vi "Camera module.vi"(8 "error in (no error)":errorcluster) -> (0 "error out":errorcluster)   [LabVIEW 2016]
uses:
  <vilib>/vision/Image Controls.llb/IMAQ Image.ctl
  <vilib>/userdefined/High Color/IMAQdx.ctl
  General/Controls/Queue modes.ctl
  General/Controls/staus modes.ctl
  Controls/Camera queue.ctl
  Controls/Camera states.ctl
  <vilib>/vision/driver/NI_Vision_Acquisition_Software.lvlib
panel:
  out "error out 2":errorcluster
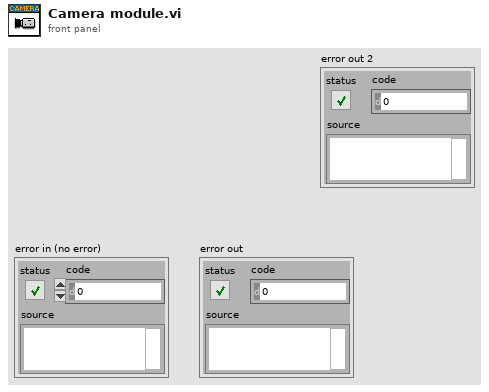
[diagram p1: front panel]
types:
  T1 = typedef "Queue modes.ctl" = enum16{"Initialise", "Destroy", "Get"}
  T2 = typedef "IMAQdx.ctl" = refnum<k21>
  T3 = typedef "IMAQ Image.ctl" = refnum<image>
  T4 = typedef "References.ctl" = cluster{"Tab Control":refnum<vi>, "Logo 1":refnum<vi>, "Logo 2":refnum<vi>, "Connect Actuator":refnum<vi>, "LIVE DATA":refnum<vi>, "Speed":refnum<vi>, "Home position":refnum<vi>, "Limit position":refnum<vi>, "Trigger":refnum<vi>, "Current position":refnum<vi>, "Connect Camera":refnum<vi>, "TEST DATA":refnum<vi>, "LIVE DATA Force":refnum<vi>, "Connect DAQ":refnum<vi>, "Initialised":refnum<vi>, "Test":refnum<vi>}
  T5 = typedef "Camera queue.ctl" = cluster{"State":T6, "Data":variant}
  T6 = typedef "Camera states.ctl" = enum16{"Initialise", "Setup", "Connect", "Snap", "Close", "Shutdown"}
  T7 = enum32{"Invalid", "Standard", "Closed", "Hidden", "Minimized", "Maximized"}
  T8 = enum8{"Enabled", "Disabled", "Disabled and Grayed Out"}
  T9 = typedef "staus modes.ctl" = enum16{"Status", "Testing", "Webcam", "DAQ", "Actuator", "Initialise"}
  T10 = cluster{"Type":u32, "Version":u32, "Flags":u32, "SerialNumberHigh":u32, "SerialNumberLow":u32, "BusType":u32, "InterfaceName":string, "VendorName":string, "ModelName":string, "CameraFileName":string, "CameraAttributeURL":string}[]
  T11 = typedef "Test settings.ctl" = cluster{"Speed (mm/s)":dbl, "Position limit":bool, "Position limit (mm)":dbl, "Load limit":bool, "Load limit (N)":dbl, "No. of repeats":u16, "Test identifier":string, "Time wait":bool, "Wait time (s)":dbl, "Trigger wait":bool, "Send trigger":bool, "Test notes":string, "Snap intervals":bool, "Time interval (s)":dbl}
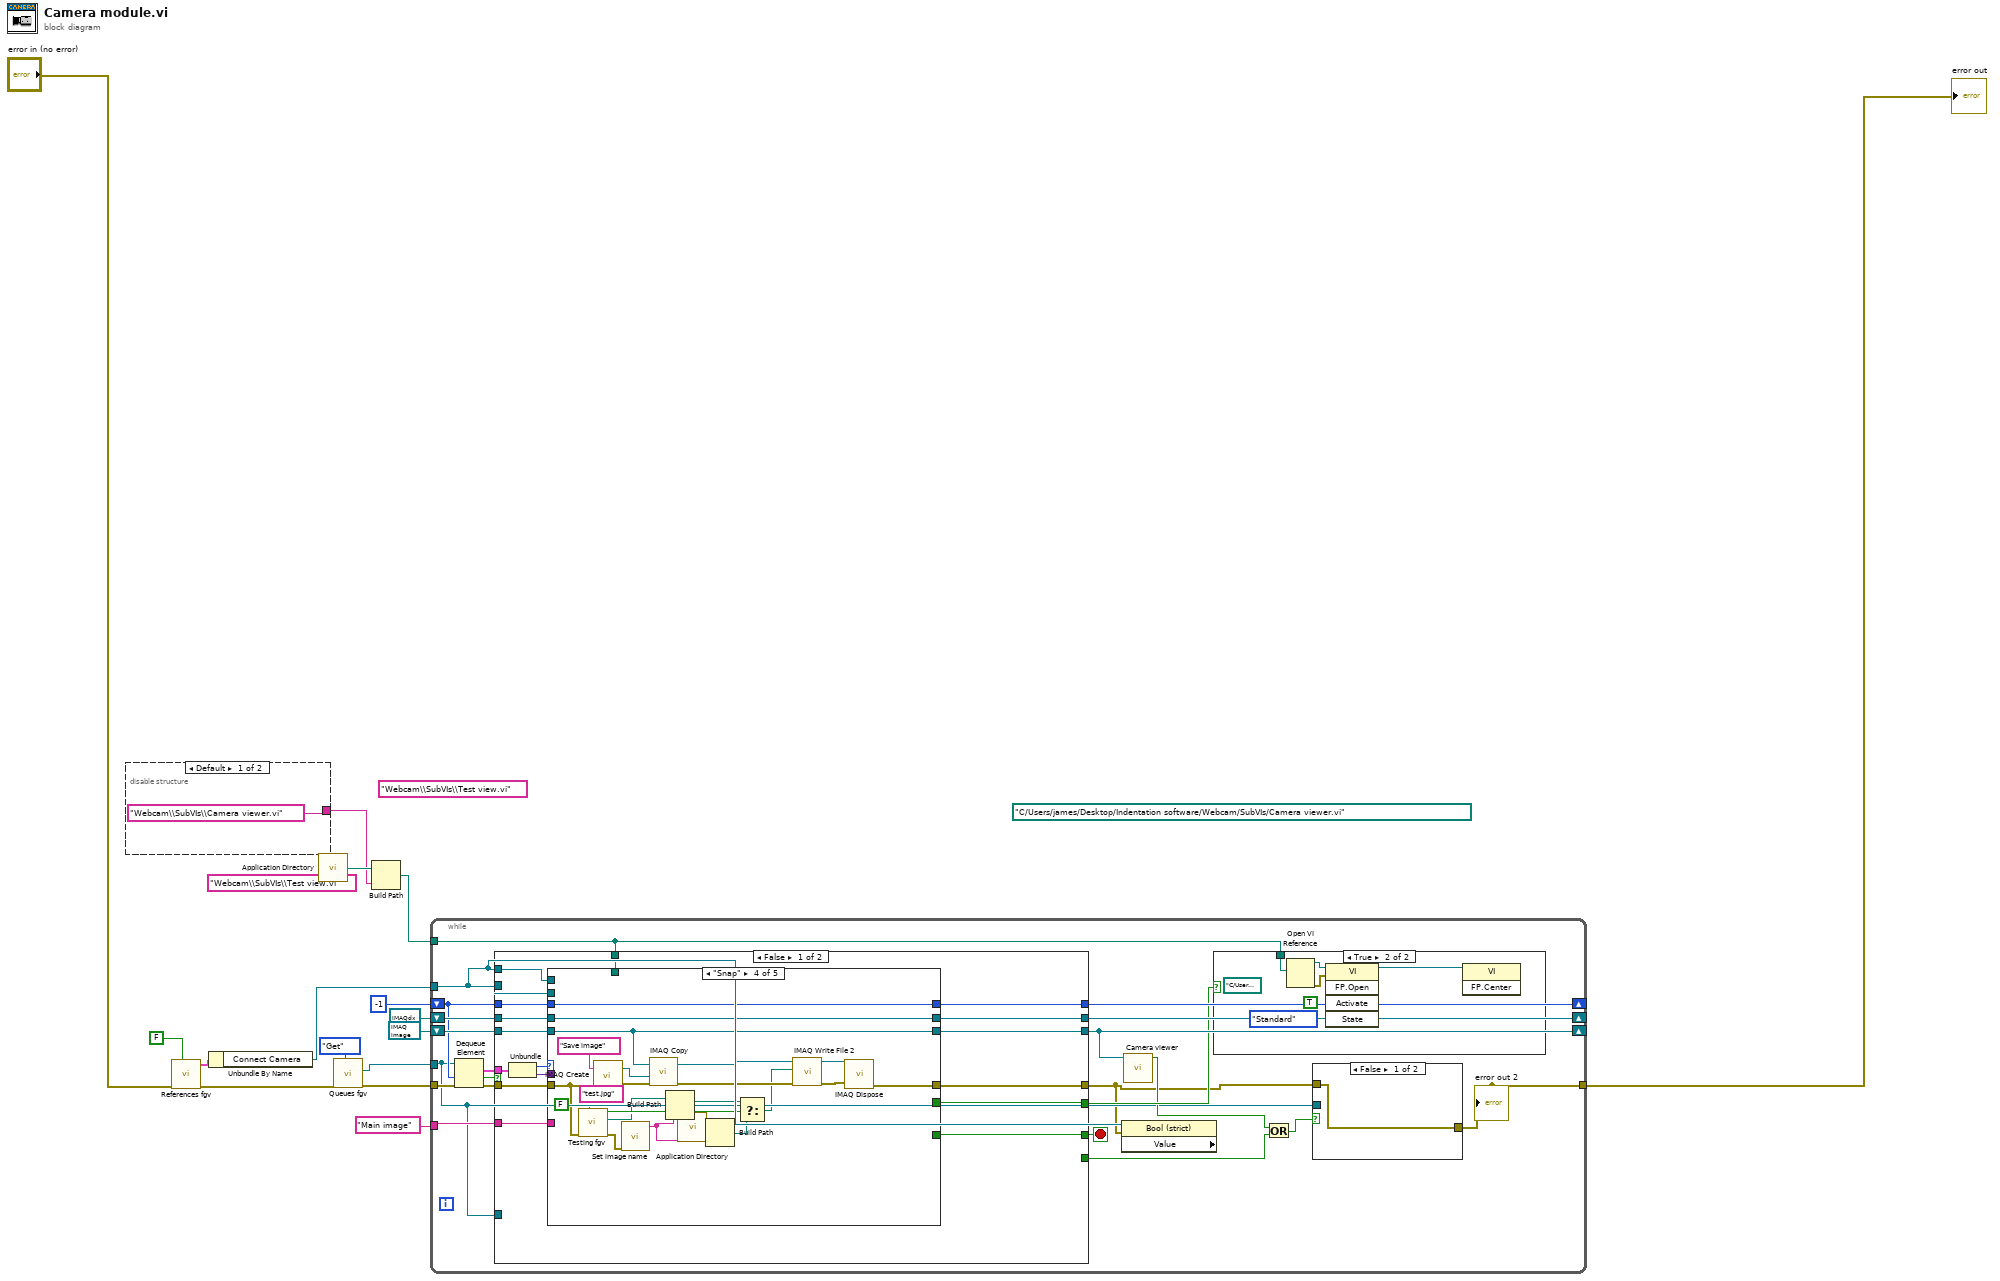
[diagram p0: block diagram]
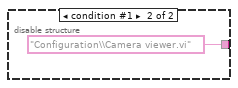
[diagram p2: hidden frame]
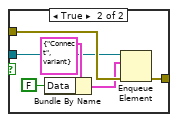
[diagram p3: hidden frame]
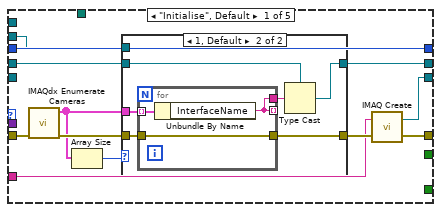
[diagram p5: hidden frame]
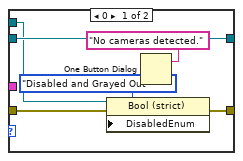
[diagram p6: hidden frame]
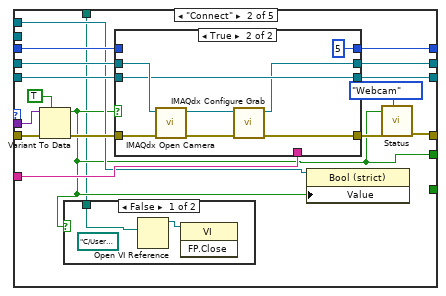
[diagram p7: hidden frame]
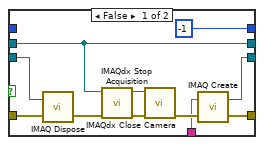
[diagram p9: hidden frame]
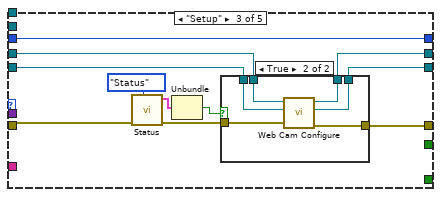
[diagram p10: hidden frame]
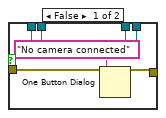
[diagram p11: hidden frame]
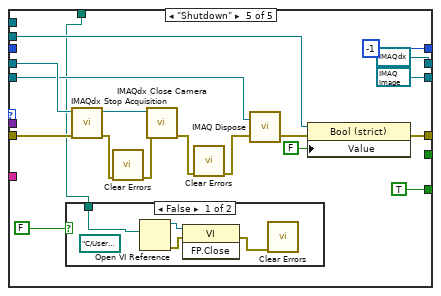
[diagram p12: hidden frame]
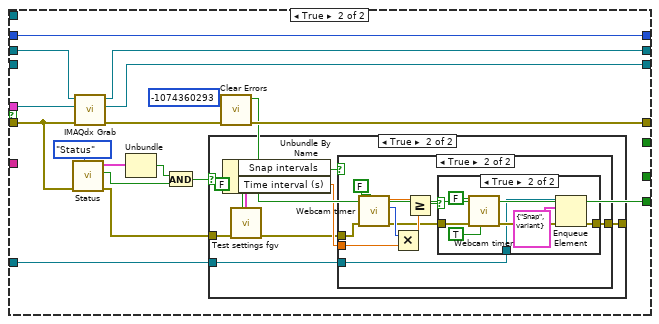
[diagram p14: hidden frame]
diagram:
  (unwired) "Webcam\\SubVIs\\Test view.vi" ("name or relative path")
  (unwired) "Webcam\\SubVIs\\Test view.vi" ("name or relative path")
  (unwired) path "C:/Users/james/Desktop/Indentation software/Webcam/SubVIs/Camera viewer.vi" ("vi path")
  n1 = disable-structure shown="Default" {
    disable-tunnel: ["Webcam\\SubVIs\\Camera viewer.vi" ("name or relative path") "Configuration\\Camera viewer.vi" ("name or relative path")] -> w1
    frame condition #0 (active) {
    }
    frame condition #1 {
    }
  }
  n2 = call "References fgv.vi"("Set?"=FALSE, "error in (no error)"="error in (no error)") -> ("error out"=w8:errorcluster, "Cluster"=w5:T4)  [unwired: 8 in]
  n3 = Unbundle By Name(w5) -> ("Connect Camera"=w4:refnum<vi>)
  n4 = call <vilib>:"Application Directory.vi"() -> ("Application Directory"=w3:path)
  n5 = call "Queues fgv.vi"("Modes"=Queue_modes."Get", "error in (no error)"=w8) -> ("error in (no error) 2"=w15:errorcluster, "Camera"=w14:refnum<queue>)  [unwired: 6 in, 2 out]
  n6 = Build Path(base path=w3, name or relative path=w1) -> (appended path=w2:path)
  n7 = while {
    tunnel: w14 -> [w21]
    tunnel: w15 -> [w39]
    tunnel: [w26] -> w13
    shift-right: [w33] -> _
    shift-left: T2 refnum ("Session Out") -> [w34]
    shift-right: [w28] -> _
    shift-left: T3 refnum ("New Image") -> [w35]
    tunnel: w4 -> [w22]
    shift-right: [w30] -> _
    shift-left: -1 ("timeout in ms (-1)") -> [w31]
    tunnel: "Main image" ("Image Name") -> [w29]
    tunnel: w2 -> [w20]
    stop <- w36 stop-if-true
    n8 = Dequeue Element(queue=w21, timeout in ms (-1)=w31, error in (no error)=w39) -> (element=w38:T5, timed out?=w32:bool, error out=w37:errorcluster)  [unwired: 1 out]
    n9 = case shown="False" w32 {
      tunnel: w38 -> [w69 _]
      tunnel: w37 -> [w68 w206]
      tunnel: [w65 _] -> w36
      tunnel: [w64 w209] -> w19
      tunnel: [w63 w212] -> w28
      tunnel: w35 -> [w62 w214]
      tunnel: w22 -> [w61 _]
      tunnel: w34 -> [w60 w215]
      tunnel: [w59 w213] -> w33
      tunnel: w31 -> [w58 w211]
      tunnel: [w57 w211] -> w30
      tunnel: w29 -> [w56 _]
      tunnel: [w55 _] -> w27
      tunnel: w22 -> [w54 _]
      tunnel: [_ w207] -> w24
      tunnel: w20 -> [w53 _]
      tunnel: w21 -> [_ w199]
      frame False {
        n10 = Unbundle(w69) -> ("State"=w67:T6, "Data"=w66:variant)
        n11 = case shown="\"Snap\"" w67 {
          tunnel: w68 -> [w76 w113 w139 w157 w189]
          tunnel: w66 -> [_ w112 _ _ _]
          tunnel: [_ _ _ _ TRUE] -> w65
          tunnel: [w81 w100 w145 w168 w193] -> w64
          tunnel: [w80 w107 w141 w171 T3 refnum ("New Image out")] -> w63
          tunnel: w62 -> [_ w108 w143 w171 w187]
          tunnel: w61 -> [w71 _ _ _ w191]
          tunnel: w60 -> [w78 w109 w144 w176 w188]
          tunnel: [w77 w106 w142 w176 T2 refnum ("Session Out out")] -> w59
          tunnel: w58 -> [w79 w105 w140 w175 _]
          tunnel: [w79 w104 w140 w175 -1 ("timeout in ms (-1)")] -> w57
          tunnel: w56 -> [w73 w103 _ _ _]
          tunnel: [_ w98 _ _ _] -> w55
          tunnel: w54 -> [_ w99 _ _ _]
          tunnel: w53 -> [_ w97 _ _ w178]
          frame "Initialise", Default {
            n12 = call <vilib>:"IMAQdx Enumerate Cameras.vi"("error in"=w76) -> ("error out"=w75:errorcluster, "Camera Information Array"=w72:T10)  [unwired: 9 in]
            n13 = Array Size(array=w72) -> (size(s)=w70:i32)
            n14 = case shown="1, Default" w70 {
              tunnel: w78 -> [w87 w93]
              tunnel: [w87 w92] -> w77
              tunnel: w75 -> [w85 w91]
              tunnel: [w83 w89] -> w74
              tunnel: w72 -> [_ w88]
              tunnel: w71 -> [w84 _]
              frame 0 {
                n15 = property class="Bool (strict)"(reference=w84, error in=w85, "DisabledEnum"=T8."Disabled and Grayed Out" ("Disabled")) -> (error out=w83:errorcluster)  [unwired: 1 out]
                n16 = One Button Dialog(message="No cameras detected.") -> ()  [unwired: 1 in, 1 out]
              }
              frame 1, Default {
                n17 = for {
                  tunnel: w88 -> [w96] mode=indexing
                  tunnel: [w95] -> _ mode=indexing
                  tunnel: [w95] -> w90
                  tunnel: w91 -> [w94]
                  tunnel: [w94] -> w89
                  n18 = Unbundle By Name(w96) -> ("InterfaceName"=w95:string)
                }
                n19 = Type Cast(type=w93, x=w90) -> (*(type *) &x=w92:T2)
              }
            }
            n20 = call "IMAQ Create"("Image Name"=w73, "error in (no error)"=w74) -> ("New Image"=w80:T3, "error out"=w81:errorcluster)  [unwired: 3 in]
          }
          frame "Connect" {
            n21 = Variant To Data(error in=w113, type=TRUE, Variant=w112) -> (data=w98:bool, error out=w110:errorcluster)
            n22 = case shown="False" w98 {
              tunnel: w97 -> [w114 _]
              frame False {
                (unwired) path "C:/Users/james/Desktop/Indentation software/Webcam/SubVIs/Camera viewer.vi" ("vi path")
                n23 = Open VI Reference(vi path=w114) -> (vi reference=w115:refnum<vi>)  [unwired: 5 in, 1 out]
                n24 = invoke class="VI" method="FP.Close"(reference=w115) -> ()  [unwired: 2 in, 3 out]
              }
              frame True {
              }
            }
            n25 = case shown="True" w98 {
              tunnel: w110 -> [w122 w134]
              tunnel: w109 -> [w123 w133]
              tunnel: w108 -> [w120 w132]
              tunnel: [w118 w128] -> w102
              tunnel: [w117 w132] -> w107
              tunnel: [w123 w127] -> w106
              tunnel: w105 -> [_ _]
              tunnel: [-1 ("timeout in ms (-1)") 5 ("timeout in ms (-1)")] -> w104
              tunnel: w103 -> [w116 _]
              frame False {
                n26 = call "IMAQ Dispose"("Image"=w120, "error in (no error)"=w122) -> ("error out"=w121:errorcluster)  [unwired: 4 in]
                n27 = call <vilib>:"IMAQdx Stop Acquisition.vi"("error in"=w121, "Session In"=w123) -> ("error out"=w125:errorcluster, "Session Out"=w126:T2)  [unwired: 8 in]
                n28 = call <vilib>:"IMAQdx Close Camera.vi"("error in"=w125, "Session In"=w126) -> ("error out"=w119:errorcluster)  [unwired: 9 in]
                n29 = call "IMAQ Create"("Image Name"=w116, "error in (no error)"=w119) -> ("New Image"=w117:T3, "error out"=w118:errorcluster)  [unwired: 3 in]
              }
              frame True {
                n30 = call <vilib>:"IMAQdx Open Camera.vi"("error in"=w134, "Session In"=w133) -> ("error out"=w129:errorcluster, "Session Out"=w130:T2)  [unwired: 1 in, 7 out]
                n31 = call <vilib>:"IMAQdx Configure Grab.vi"("error in"=w129, "Session In"=w130) -> ("error out"=w128:errorcluster, "Session Out"=w127:T2)  [unwired: 8 in]
              }
            }
            n32 = property class="Bool (strict)"(reference=w99, "Value"=w98) -> ()  [unwired: 1 in, 2 out]
            n33 = call "Status.vi"("Mode"=staus_modes."Webcam", "error in (no error)"=w102, "Data"=w98) -> ("error out"=w100:errorcluster)  [unwired: 6 in, 2 out]
          }
          frame "Setup" {
            n34 = call "Status.vi"("Mode"=staus_modes."Status", "error in (no error)"=w139) -> ("error out"=w138:errorcluster, "Connections"=w136:cluster{"Data":bool, "Data":bool, "Data":bool})  [unwired: 7 in, 1 out]
            n35 = Unbundle(w136) -> ("Data"=w135:bool)  [unwired: 2 out]
            n36 = case shown="True" w135 {
              tunnel: [w147 w155] -> w145
              tunnel: w144 -> [w148 w154]
              tunnel: w143 -> [w149 w153]
              tunnel: [w148 w152] -> w142
              tunnel: [w149 w151] -> w141
              tunnel: w138 -> [w147 w150]
              frame False {
                n37 = One Button Dialog(message="No camera connected") -> ()  [unwired: 1 in, 1 out]
              }
              frame True {
                n38 = call "Web Cam Configure.vi"("error in (no error)"=w150, "New Image in"=w153, "Session Cam In"=w154) -> ("error out"=w155:errorcluster, "New Image out"=w151:T3, "Session Out out"=w152:T2)  [unwired: 6 in]
              }
            }
          }
          frame "Snap" {
            (unwired) "test.jpg" ("name or relative path")
            n39 = call "Testing fgv.vi"("Populate"=FALSE, "error in (no error)"=w157) -> ("error out"=w161:errorcluster, "test dir"=w164:path, "Testing?"=w165:bool)  [unwired: 7 in]
            n40 = call "IMAQ Create"("Image Name"="Save image", "error in (no error)"=w157) -> ("New Image"=w172:T3, "error out"=w173:errorcluster)  [unwired: 3 in]
            n41 = call "Set image name.vi"("error in (no error)"=w161) -> ("image name"=w160:string)  [unwired: 9 in, 1 out]
            n42 = call "IMAQ Copy"("error in (no error)"=w173, "Image Dst"=w172, "Image Src"=w171) -> ("error out"=w170:errorcluster, "Image Dst Out"=w169:T3)  [unwired: 3 in]
            n43 = Build Path(base path=w164, name or relative path=w160) -> (appended path=w163:path)
            n44 = call <vilib>:"Application Directory.vi"() -> ("Application Directory"=w158:path)
            n45 = Build Path(base path=w158, name or relative path=w160) -> (appended path=w159:path)
            n46 = Select(t=w163, s=w165, f=w159) -> (s? t:f=w162:path)
            n47 = call-poly "IMAQ Write File 2"("error in (no error)"=w170, "File Path"=w162, "Image"=w169) -> ("error out"=w167:errorcluster, "Image Out (duplicate)"=w166:T3)  [unwired: 7 in]
            n48 = call "IMAQ Dispose"("Image"=w166, "error in (no error)"=w167) -> ("error out"=w168:errorcluster)  [unwired: 4 in]
          }
          frame "Shutdown" {
            n49 = case shown="False" FALSE {
              tunnel: w178 -> [w197 _]
              frame False {
                (unwired) path "C:/Users/james/Desktop/Indentation software/Webcam/SubVIs/Camera viewer.vi" ("vi path")
                n50 = Open VI Reference(vi path=w197) -> (vi reference=w198:refnum<vi>, error out=w196:errorcluster)  [unwired: 5 in]
                n51 = invoke class="VI" method="FP.Close"(reference=w198, error in=w196) -> (error out=w195:errorcluster)  [unwired: 1 in, 2 out]
                n52 = call <vilib>:"Clear Errors.vi"("error in (no error)"=w195) -> ()  [unwired: 5 in, 2 out]
              }
              frame True {
              }
            }
            n53 = call <vilib>:"IMAQdx Stop Acquisition.vi"("error in"=w189, "Session In"=w188) -> ("error out"=w182:errorcluster, "Session Out"=w190:T2)  [unwired: 8 in]
            n54 = call <vilib>:"Clear Errors.vi"("error in (no error)"=w182) -> ("error out"=w181:errorcluster)  [unwired: 5 in, 1 out]
            n55 = call <vilib>:"IMAQdx Close Camera.vi"("error in"=w181, "Session In"=w190) -> ("error out"=w180:errorcluster)  [unwired: 9 in]
            n56 = call <vilib>:"Clear Errors.vi"("error in (no error)"=w180) -> ("error out"=w179:errorcluster)  [unwired: 5 in, 1 out]
            n57 = call "IMAQ Dispose"("Image"=w187, "error in (no error)"=w179) -> ("error out"=w186:errorcluster)  [unwired: 4 in]
            n58 = property class="Bool (strict)"(reference=w191, error in=w186, "Value"=FALSE) -> (error out=w193:errorcluster)  [unwired: 1 out]
          }
        }
      }
      frame True {
        n59 = call "Status.vi"("Mode"=staus_modes."Status", "error in (no error)"=w206) -> ("error out"=w200:errorcluster, "Testing"=w202:bool, "Connections"=w204:cluster{"Data":bool, "Data":bool, "Data":bool})  [unwired: 7 in]
        n60 = call <vilib>:"IMAQdx Grab.vi"("error in"=w206, "Image In"=w214, "Session In"=w215) -> ("error out"=w210:errorcluster, "Image Out"=w212:T3, "Session Out"=w213:T2)  [unwired: 1 in, 5 out]
        n61 = Unbundle(w204) -> ("Data"=w203:bool)  [unwired: 2 out]
        n62 = And(x=w203, y=w202) -> (x .and. y?=w201:bool)
        n63 = case shown="True" w201 {
          tunnel: w200 -> [_ w220]
          tunnel: [_ w218] -> _
          tunnel: w199 -> [_ w217]
          frame False {
          }
          frame True {
            n64 = call "Test settings fgv.vi"("Set?"=FALSE, "error in (no error)"=w220) -> ("error out"=w216:errorcluster, "Test settings out"=w222:T11)  [unwired: 7 in, 1 out]
            n65 = Unbundle By Name(w222) -> ("Snap intervals"=w221:bool, "Time interval (s)"=w219:dbl)
            n66 = case shown="True" w221 {
              tunnel: w219 -> [_ w231]
              tunnel: [_ w226] -> w218
              tunnel: w217 -> [_ w225]
              tunnel: w216 -> [_ w224]
              frame False {
              }
              frame True {
                n67 = call "Webcam timer.vi"("Reset"=FALSE, "error in (no error)"=w224) -> ("error out"=w227:errorcluster, "Int"=w232:i32, "Time"=w230:dbl)  [unwired: 7 in]
                n68 = Multiply(x=w232, y=w231) -> (x*y=w229:dbl)
                n69 = Greater Or Equal?(x=w230, y=w229) -> (x >= y?=w228:bool)
                n70 = case shown="True" w228 {
                  tunnel: w227 -> [_ w238]
                  tunnel: [_ w236] -> w226
                  tunnel: w225 -> [_ w235]
                  frame False {
                  }
                  frame True {
                    n71 = call "Webcam timer.vi"("Inc?"=TRUE, "Reset"=FALSE, "error in (no error)"=w238) -> ("error out"=w237:errorcluster)  [unwired: 6 in, 2 out]
                    n72 = Enqueue Element(queue=w235, element=T5 {"State"=enum."Snap", "Data"=variant}, error in (no error)=w237) -> (error out=w236:errorcluster)  [unwired: 1 in, 2 out]
                  }
                }
              }
            }
          }
        }
        n73 = call <vilib>:"Clear Errors.vi"("error in (no error)"=w210, "specific error code to clear (0: all)"=-1074360293) -> ("error out"=w209:errorcluster, "specific error cleared?"=w207:bool)  [unwired: 4 in]
      }
    }
    n74 = property class="Bool (strict)" props=["Value"](reference=w22, error in=w19) -> ()  [unwired: 3 out]
    n75 = call "Camera viewer.vi"("CAMERA FEED 2"=w28) -> ("Closed"=w25:bool)  [unwired: 10 in]
    n76 = case shown="True" w27 {
      tunnel: w20 -> [_ w48]
      frame False {
      }
      frame True {
        (unwired) path "C:/Users/james/Desktop/Indentation software/Webcam/SubVIs/Camera viewer.vi" ("vi path")
        n77 = Open VI Reference(vi path=w48) -> (vi reference=w51:refnum<vi>, error out=w52:errorcluster)  [unwired: 5 in]
        n78 = invoke class="VI" method="FP.Open"(reference=w51, error in=w52, "Activate"=TRUE ("Activate?"), "State"=T7."Standard") -> (reference out=w47:refnum<vi>)  [unwired: 1 in, 4 out]
        n79 = invoke class="VI" method="FP.Center"(reference=w47) -> ()  [unwired: 2 in, 3 out]
      }
    }
    n80 = Or(x=w25, y=w24) -> (x .or. y?=w23:bool)
    n81 = case shown="False" w23 {
      tunnel: w19 -> [w40 w45]
      tunnel: [w40 w44] -> w26
      tunnel: w21 -> [_ w42]
      frame False {
      }
      frame True {
        n82 = Bundle By Name(cluster=T5 {"State"=enum."Connect", "Data"=variant}, "Data"=FALSE) -> (w43:T5)
        n83 = Enqueue Element(queue=w42, element=w43, error in (no error)=w45) -> (error out=w44:errorcluster)  [unwired: 1 in, 2 out]
      }
    }
    "error out 2" <- w26
  }
  "error out" <- w13
